vi "UI References Queue FGV.vi"(8 "error in (no error)":errorcluster, 9 "Action (\"Get References\")":T2=enum."Get References", 11 "UI References in":T1) -> (0 "error out":errorcluster, 3 "UI References out":T1)   [LabVIEW 2018, in "Numeric Data Type.lvclass"]
uses:
  Numeric Data Type.lvclass
  UI References Queue FGV Actions Enum.ctl
  UI References.ctl
  Representation Ring.ctl
  <vilib>/fxp/FXPxcontrol/FXP.xctl
  Response to Values Outside of Limits Enum.ctl
  Precision Type.ctl
  Padding.ctl
  Time Format.ctl
  Clock Type.ctl
  Date Format.ctl
  Date Order.ctl
  Year Format.ctl
  Format Code Type List Enum.ctl
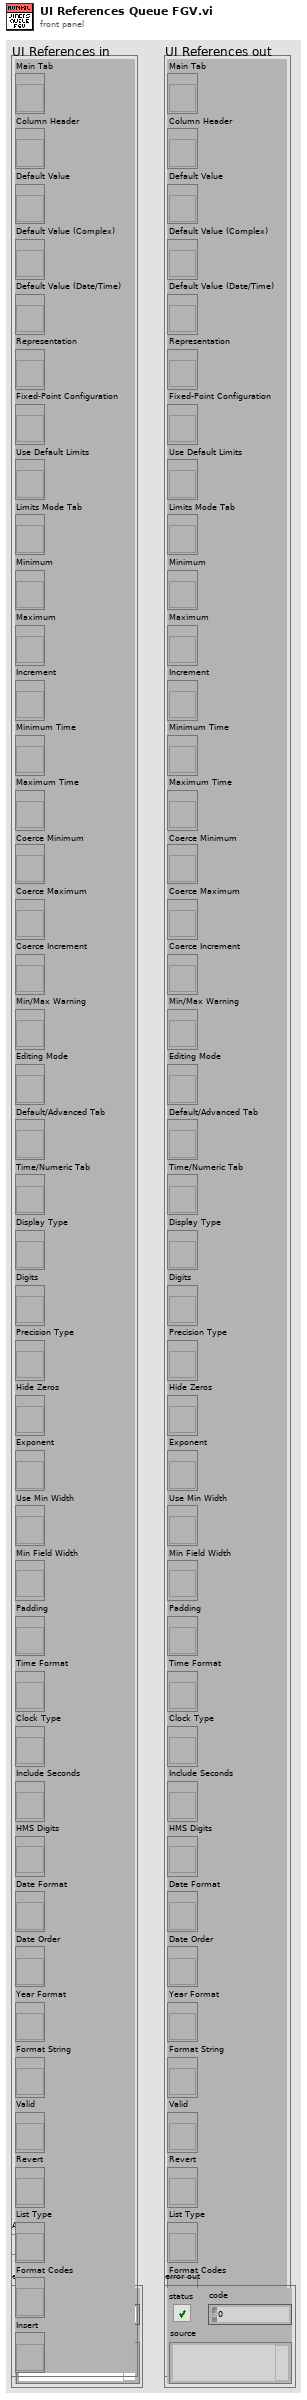
[diagram p1: front panel]
types:
  T1 = typedef "Numeric Data Type.lvclass/UI References.ctl" = cluster{"Main Tab":refnum<vi>, "Column Header":refnum<vi>, "Default Value":refnum<vi>, "Default Value (Complex)":refnum<vi>, "Default Value (Date/Time)":refnum<vi>, "Representation":refnum<vi>, "Fixed-Point Configuration":refnum<vi>, "Use Default Limits":refnum<vi>, "Limits Mode Tab":refnum<vi>, "Minimum":refnum<vi>, "Maximum":refnum<vi>, "Increment":refnum<vi>, "Minimum Time":refnum<vi>, "Maximum Time":refnum<vi>, "Coerce Minimum":refnum<vi>, "Coerce Maximum":refnum<vi>, "Coerce Increment":refnum<vi>, "Min/Max Warning":refnum<vi>, "Editing Mode":refnum<vi>, "Default/Advanced Tab":refnum<vi>, "Time/Numeric Tab":refnum<vi>, "Display Type":refnum<vi>, "Digits":refnum<vi>, "Precision Type":refnum<vi>, "Hide Zeros":refnum<vi>, "Exponent":refnum<vi>, "Use Min Width":refnum<vi>, "Min Field Width":refnum<vi>, "Padding":refnum<vi>, "Time Format":refnum<vi>, "Clock Type":refnum<vi>, "Include Seconds":refnum<vi>, "HMS Digits":refnum<vi>, "Date Format":refnum<vi>, "Date Order":refnum<vi>, "Year Format":refnum<vi>, "Format String":refnum<vi>, "Valid":refnum<vi>, "Revert":refnum<vi>, "List Type":refnum<vi>, "Format Codes":refnum<vi>, "Insert":refnum<vi>}
  T2 = typedef "Numeric Data Type.lvclass/UI References Queue FGV Actions Enum.ctl" = enum16{"Initialize References", "Get References"}
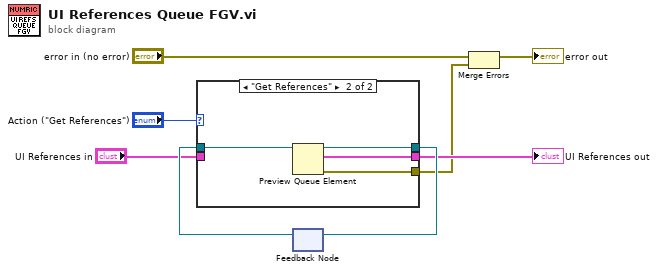
[diagram p0: block diagram]
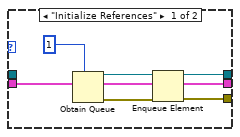
[diagram p2: hidden frame]
diagram:
  n1 = feedback #1() -> (w6:refnum<queue>)  [unwired: 1 in]
  n2 = case shown="\"Get References\"" "Action (\"Get References\")" {
    tunnel: [w11 w17] -> w7
    tunnel: w6 -> [_ w18]
    tunnel: [w9 w16] -> w5
    tunnel: [w10 w15] -> w4
    tunnel: "UI References in" -> [w9 _]
    frame "Initialize References" {
      n3 = Obtain Queue(max queue size (-1, unlimited)=1, element data type=w9) -> (queue out=w13:refnum<queue>, error out=w12:errorcluster)  [unwired: 3 in, 1 out]
      n4 = Enqueue Element(queue=w13, element=w9, error in (no error)=w12) -> (queue out=w11:refnum<queue>, error out=w10:errorcluster)  [unwired: 1 in, 1 out]
    }
    frame "Get References" {
      n5 = Preview Queue Element(queue=w18) -> (queue out=w17:refnum<queue>, element=w16:T1, error out=w15:errorcluster)  [unwired: 2 in, 1 out]
    }
  }
  "UI References out" <- w5
  n6 = feedback-in #1(w7) -> ()
  n7 = Merge Errors("error in (no error)", w4) -> (→"error out":errorcluster)
